vi "Increment Progress Bar.vi"(8 "error in (no error)":errorcluster, 10 "Step Name (\"\")":string, 11 "Progress Bar Dialog in":refnum<class "Progress Bar Dialog.lvclass">) -> (0 "error out":errorcluster, 2 "Cancelled?":bool, 3 "Progress Bar Dialog out":refnum<class "Progress Bar Dialog.lvclass">)   [LabVIEW 2020, in "Progress Bar Dialog.lvclass"]
doc: "Calling this function will increment the progress bar by one. The optional input for 'Step Name' allows you to display text for the current item."
uses:
  <vilib>/ProgressBar/Progress Bar Dialog.lvclass
  <vilib>/ProgressBar/Progress Bar Dialog.lvclass/Progress Bar Dialog.ctl
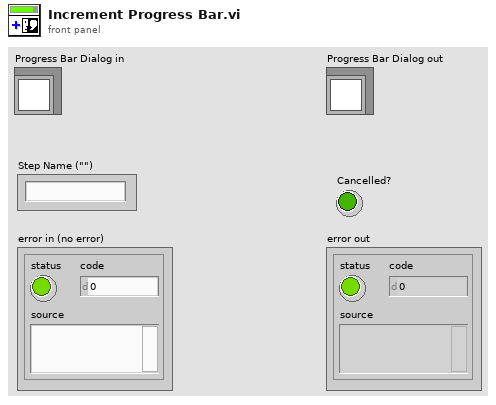
[diagram p1: front panel]
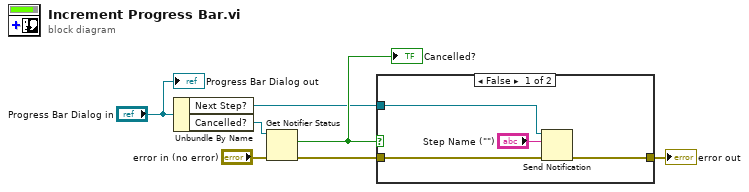
[diagram p0: block diagram]
diagram:
  n1 = Unbundle By Name("Progress Bar Dialog in") -> ("Next Step?"=w1:refnum<notifier>, "Cancelled?"=w6:refnum<notifier>)
  n2 = Get Notifier Status(notifier=w6, error in (no error)="error in (no error)") -> (current notification=w5:bool, error out=w3:errorcluster)  [unwired: 3 out]
  "Cancelled?" <- w5
  n3 = case shown="False" w5 {
    tunnel: w1 -> [w10 _]
    tunnel: w3 -> [w9 w12]
    tunnel: [w8 w12] -> w2
    frame False {
      n4 = Send Notification(notification="Step Name (\"\")", notifier=w10, error in (no error)=w9) -> (error out=w8:errorcluster)  [unwired: 1 out]
    }
    frame True {
    }
  }
  "error out" <- w2
  "Progress Bar Dialog out" <- "Progress Bar Dialog in"
